vi "Launcher Preperation.vi"(2 "Elevation":dbl, 3 "Shooting Motors":dbl, 4 "Auto Shoot":bool) -> (1 "READY!":bool)   [LabVIEW 2012]
uses:
  Motors Values.vi
  BotStatus.vi
  <vilib>/express/express arith-compare/Formula/XNode/ExpressFormulaBlockNode.xnode
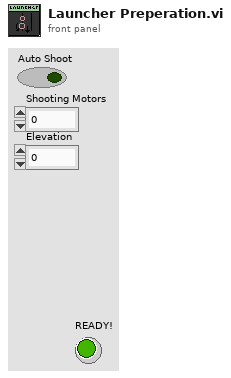
[diagram p1: front panel]
types:
  T1 = cluster{"Middle":bool, "InCannon":bool, "InFlipper":bool, "FlipperAtPlace":bool, "Bottom":bool, "FrisbeeDirection":bool}
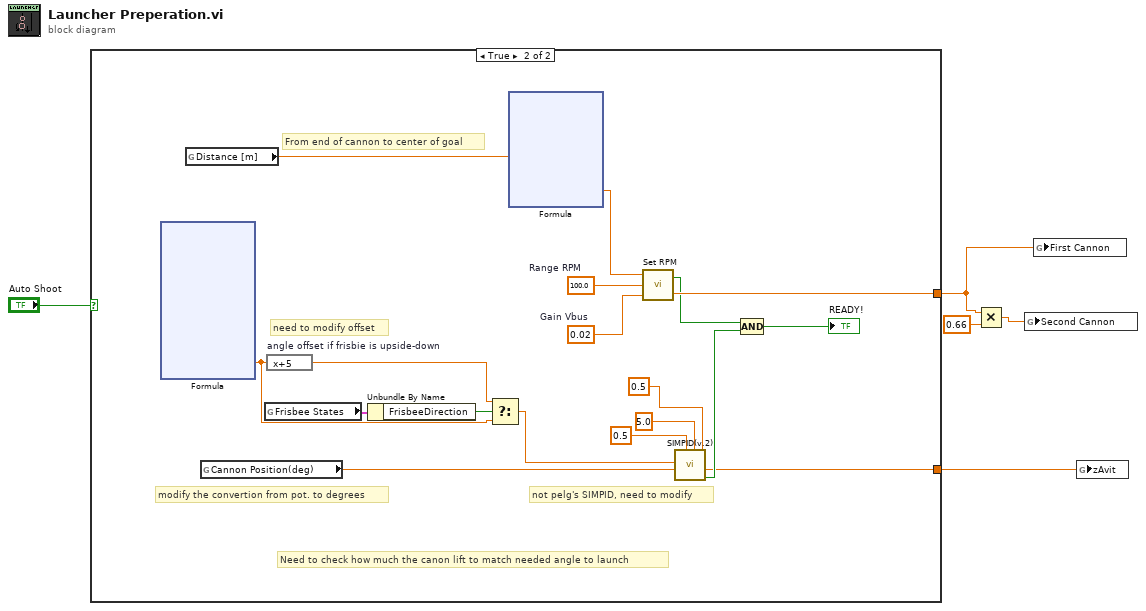
[diagram p0: block diagram]
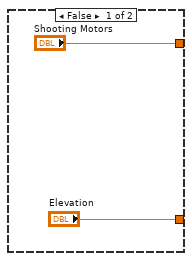
[diagram p2: hidden frame]
diagram:
  n1 = case shown="True" "Auto Shoot" {
    tunnel: ["Elevation" w13] -> w3
    tunnel: ["Shooting Motors" w11] -> w2
    frame False {
    }
    frame True {
      w8 = 0.02  # Gain Vbus
      w9 = 100.0  # Range RPM
      # "From end of cannon to center of goal"
      # "need to modify offset"
      # "not pelg's SIMPID, need to modify"
      # "modify the convertion from pot. to degrees"
      # "Need to check how much the canon lift to match needed angle to launch"
      n2 = xnode "Formula"() -> ("Result"=w19:dbl)  [unwired: 5 in, 1 out]
      n3 = global read "BotStatus.vi" "Distance [m]"() -> (w16:dbl)
      n4 = global read "BotStatus.vi" "Cannon Position(deg)"() -> (w17:dbl)
      n5 = global read "BotStatus.vi" "Frisbee States"() -> (w15:T1)
      n6 = expression code="x+5" "angle offset if frisbie is upside-down"(w19) -> (w18:dbl)
      n7 = Unbundle By Name(w15) -> ("FrisbeeDirection"=w14:bool)
      n8 = Select(t=w18, s=w14, f=w19) -> (s? t:f=w20:dbl)
      n9 = xnode "Formula"("D"=w16) -> ("Result"=w12:dbl)  [unwired: 2 in, 1 out]
      n10 = call "Set RPM.vi"("Gain Vbus"=w8, "Range RPM"=w9, "Set Point RPM"=w12) -> ("Vbus Out"=w11:dbl, "READY!"=w10:bool)
      n11 = call "SIMPID(v.2).vi"("Range"=0.5, "upper limit"=5.0, "lower limit"=0.5, "Current Point"=w17, "Set Point"=w20) -> ("On Target"=w24:bool, "result"=w13:dbl)  [unwired: 5 in]
      n12 = Compound Arithmetic op=AND(w10, w24) -> (→"READY!":bool)
    }
  }
  n13 = Multiply(x=w2, y=0.66) -> (x*y=w4:dbl)
  n14 = global write "Motors Values.vi" "Second Cannon"(w4) -> ()
  n15 = global write "Motors Values.vi" "First Cannon"(w2) -> ()
  n16 = global write "Motors Values.vi" "zAvit"(w3) -> ()
